vi "test_SetItemInfoDependencies_TargetsDifferentCompilersAdvancedPPLSolution.vi"() -> (3 "Pass?":bool)   [LabVIEW 2019, in "Tests.SolutionBuilder.lvlib"]
uses:
  Tests.SolutionBuilder.lvlib
  SolutionBuilder/SolutionBuilder.lvclass
  SolutionBuilder/ProjectItem/ProjectItem.lvclass
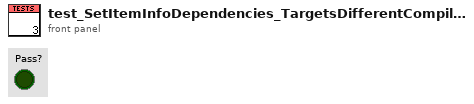
[diagram p1: front panel]
types:
  T1 = cluster{"Relative Path from 1 to 2":path, string[]}
  T2 = cluster{"Relative Path from 1 to 2":path, "appended array":string[]}
  T3 = cluster{"Relative Path from 1 to 2":path, "appended array":string[]}[]
  T4 = cluster{"Relative Path from 1 to 2":path, string[]}[]
  T5 = typedef "SolutionBuilder.lvlib/SolutionBuilder.lvclass/ProjectItemMap.ctl" = map{path, refnum<class "ProjectItem.lvclass">[]}
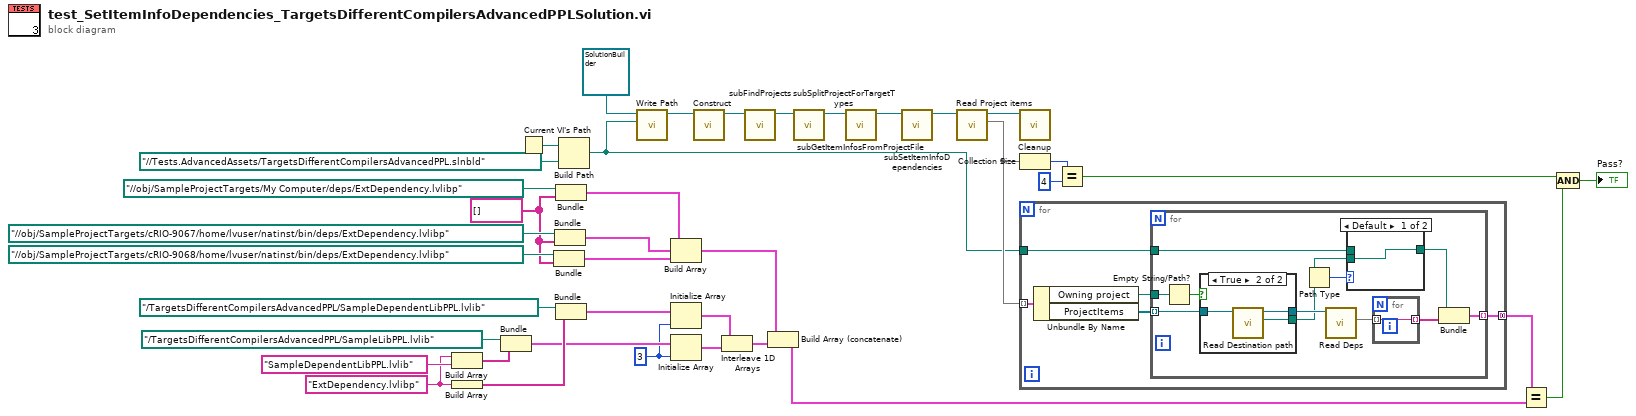
[diagram p0: block diagram]
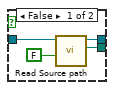
[diagram p2: hidden frame]
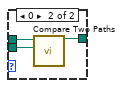
[diagram p3: hidden frame]
diagram:
  w6 = string[] [] ("appended array")
  w15 = 3 ("dimension size")
  w23 = "ExtDependency.lvlibp"
  n1 = Build Array(w23, "SampleDependentLibPPL.lvlib") -> (w18:string[])
  n2 = Build Array(w23) -> (w20:string[])
  n3 = Bundle("Relative Path from 1 to 2"=path "../TargetsDifferentCompilersAdvancedPPL/SampleLibPPL.lvlib", w18) -> (w16:T1)  [unwired: 1 in]
  n4 = Current VI's Path() -> (path=w38:path)
  n5 = Bundle("Relative Path from 1 to 2"=path "../../obj/SampleProjectTargets/cRIO-9068/home/lvuser/natinst/bin/deps/ExtDependency.lvlibp", "appended array"=w6) -> (w5:T2)  [unwired: 1 in]
  n6 = Bundle("Relative Path from 1 to 2"=path "../../obj/SampleProjectTargets/cRIO-9067/home/lvuser/natinst/bin/deps/ExtDependency.lvlibp", "appended array"=w6) -> (w4:T2)  [unwired: 1 in]
  n7 = Bundle("Relative Path from 1 to 2"=path "../../obj/SampleProjectTargets/My Computer/deps/ExtDependency.lvlibp", "appended array"=w6) -> (w10:T2)  [unwired: 1 in]
  n8 = Bundle("Relative Path from 1 to 2"=path "../TargetsDifferentCompilersAdvancedPPL/SampleDependentLibPPL.lvlib", w20) -> (w17:T1)  [unwired: 1 in]
  n9 = Build Path(base path=w38, name or relative path=path "../../Tests.AdvancedAssets/TargetsDifferentCompilersAdvancedPPL.slnbld" ("Path")) -> (appended path=w26:path)
  n10 = call "Write Path.vi"("Path"=w26, "SolutionBuilder in"=refnum<class "SolutionBuilder.lvclass"> refnum) -> ("SolutionBuilder out"=w30:refnum<class "SolutionBuilder.lvclass">)  [unwired: 9 in]
  n11 = Build Array(w10, w4, w5) -> (w9:T3)
  n12 = Initialize Array(w17, w15) -> (w14:T4)
  n13 = Initialize Array(w16, w15) -> (w13:T4)
  n14 = call "Construct.vi"("SolutionBuilder in"=w30) -> ("SolutionBuilder out"=w29:refnum<class "SolutionBuilder.lvclass">)  [unwired: 9 in, 1 out]
  n15 = Interleave 1D Arrays(w14, w13) -> (w12:T4)
  n16 = call "subFindProjects.vi"("SolutionBuilder in"=w29) -> ("SolutionBuilder out"=w2:refnum<class "SolutionBuilder.lvclass">)  [unwired: 9 in, 1 out]
  n17 = Build Array (concatenate)(w9, w12) -> (w11:T3)
  n18 = call "subSplitProjectForTargetTypes.vi"("SolutionBuilder in"=w2) -> ("SolutionBuilder out"=w1:refnum<class "SolutionBuilder.lvclass">)  [unwired: 9 in, 1 out]
  n19 = call "subGetItemInfosFromProjectFile.vi"("SolutionBuilder in"=w1) -> ("SolutionBuilder out"=w32:refnum<class "SolutionBuilder.lvclass">)  [unwired: 9 in, 1 out]
  n20 = call "subSetItemInfoDependencies.vi"("SolutionBuilder in"=w32) -> ("SolutionBuilder out"=w31:refnum<class "SolutionBuilder.lvclass">)  [unwired: 9 in, 1 out]
  n21 = call "Read Project items.vi"("SolutionBuilder in"=w31) -> ("Project items"=w34:T5, "SolutionBuilder out"=w28:refnum<class "SolutionBuilder.lvclass">)  [unwired: 9 in]
  n22 = call "Cleanup.vi"("SolutionBuilder in"=w28) -> ()  [unwired: 9 in, 2 out]
  n23 = Collection Size(1:w34) -> (0:w36:i32)
  n24 = for {
    tunnel: w34 -> [w44] mode=indexing
    tunnel: [w42] -> w25 mode=concatenating
    tunnel: w26 -> [w41]
    n25 = Unbundle By Name(w44) -> ("Owning project"=w40:path, "ProjectItems"=w43:refnum<class "ProjectItem.lvclass">[])
    n26 = for {
      tunnel: w43 -> [w52] mode=indexing
      tunnel: [w53] -> w42 mode=indexing
      tunnel: w41 -> [w47]
      tunnel: w40 -> [w46]
      n27 = Empty String/Path?(string/path=w46) -> (empty?=w45:bool)
      n28 = case shown="True" w45 {
        tunnel: w52 -> [w59 w62]
        tunnel: [w58 w61] -> w51
        tunnel: [w56 w60] -> w49
        frame False {
          n29 = call "Read Source path.vi"("Force abs path? (T)"=FALSE, "ProjectItem in"=w59) -> ("Source path"=w56:path, "ProjectItem out"=w58:refnum<class "ProjectItem.lvclass">)  [unwired: 8 in]
        }
        frame True {
          n30 = call "Read Destination path.vi"("ProjectItem in"=w62) -> ("Destination path"=w60:path, "ProjectItem out"=w61:refnum<class "ProjectItem.lvclass">)  [unwired: 9 in]
        }
      }
      n31 = Path Type(1:w49) -> (0:w50:i16)
      n32 = call "Read Deps.vi"("ProjectItem in"=w51) -> ("Deps"=w55:set{string})  [unwired: 9 in, 1 out]
      n33 = case shown="Default" w50 {
        tunnel: w49 -> [w63 w64]
        tunnel: [w63 w66] -> w48
        tunnel: w47 -> [_ w65]
        frame Default {
        }
        frame 0 {
          n34 = call <vilib>:"Compare Two Paths.vi"("Path 2"=w64, "Path 1"=w65) -> ("Relative Path from 1 to 2"=w66:path)  [unwired: 6 in, 3 out]
        }
      }
      n35 = for {
        tunnel: w55 -> [w67] mode=indexing
        tunnel: [w67] -> w54 mode=indexing
      }
      n36 = Bundle("Relative Path from 1 to 2"=w48, w54) -> (w53:T1)  [unwired: 1 in]
    }
  }
  n37 = Equal?(x=w36, y=4) -> (x = y?=w33:bool)
  n38 = Equal?(x=w25, y=w11) -> (x = y?=w27:bool)
  n39 = Compound Arithmetic op=AND(w33, w27) -> (→"Pass?":bool)
